vi "SO2 MFR age.vi"(9 "SO2 conc":dbl=0.1, 10 "SO2 PV":dbl, 11 "Flow rate":dbl) -> (3 "SO2 MFR":dbl)   [LabVIEW 2011]
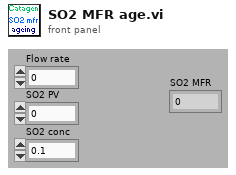
[diagram p1: front panel]
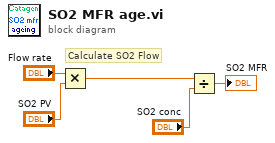
[diagram p0: block diagram]
diagram:
  # "Calculate SO2 Flow"
  n1 = Multiply(x="Flow rate", y="SO2 PV") -> (x*y=w1:dbl)
  n2 = Divide(x=w1, y="SO2 conc") -> (x/y=→"SO2 MFR":dbl)
